vi "Error Query.vi"(8 "error in (no error)":errorcluster, 11 "VISA resource name":refnum<visa-resource-name>) -> (0 "error out":errorcluster, 1 "Error Message":string, 2 "Error Code":i32[](array[numeric]), 3 "VISA resource name out":refnum<visa-resource-name>)   [LabVIEW 2020, in "BDAQ-6104.lvlib"]
doc: "Queries the instrument for any errors in the instrument's error queue. It will continue to read errors until all errors have been read from the instrument. Any errors will be returned in the <B>error out</B> control.\n\n<B>Note:</B>\nThis VI is called automatically by most driver VIs so it is not usually necessary to call this in an application."
uses:
  <instrlib>/BDAQ-6104/BDAQ-6104.lvlib
panel:
  # "EDIT: Note: The Error Query VI is included as a subVI in all driver VIs except low-level API VIs. If the instrument does not support error query, then remove the VI and remove subVI calls in each instrument driver VI that calls it."
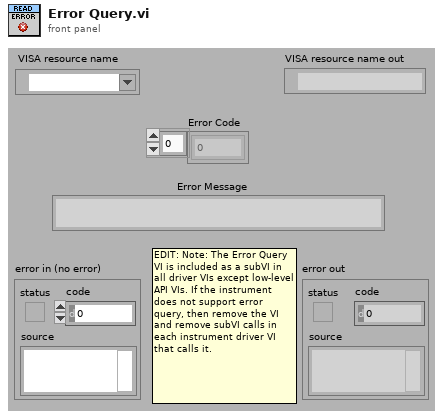
[diagram p1: front panel]
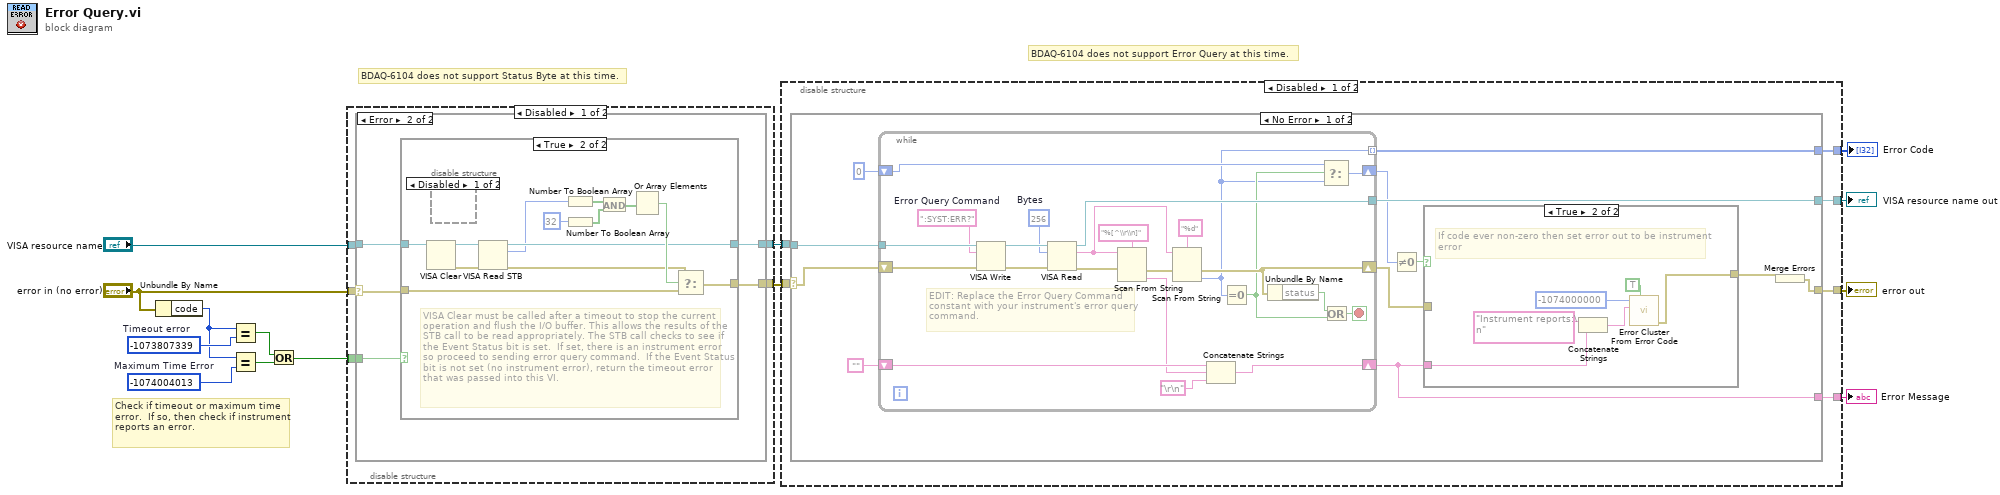
[diagram p0: block diagram]
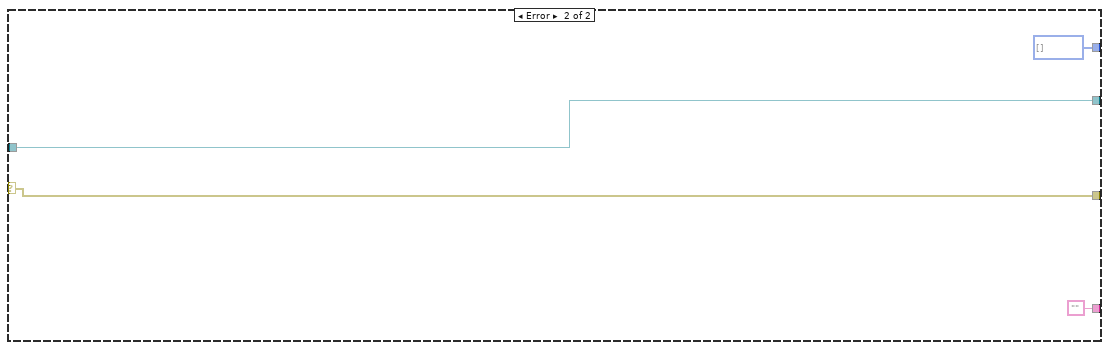
[diagram p7: hidden frame]
diagram:
  w5 = -1074004013  # Maximum Time Error
  w7 = -1073807339  # Timeout error
  # "BDAQ-6104 does not support Status Byte at this time."
  # "BDAQ-6104 does not support Error Query at this time."
  # "Check if timeout or maximum time error.  If so, then check if instrument reports an error."
  n1 = Unbundle By Name("error in (no error)") -> ("code"=w6:i32)
  n2 = Equal?(x=w6, y=w7) -> (x = y?=w3:bool)
  n3 = Equal?(x=w6, y=w5) -> (x = y?=w4:bool)
  n4 = Or(x=w3, y=w4) -> (x .or. y?=w2:bool)
  n5 = disable-structure shown="Disabled" {
    disable-tunnel: [w19 w42] -> w10
    disable-tunnel: [w18 w43] -> w9
    disable-tunnel: "VISA resource name" -> [w17 w43]
    disable-tunnel: w2 -> [w16 _]
    disable-tunnel: "error in (no error)" -> [w15 w42]
    frame Disabled {
      n6 = case shown="Error" w15 {
        selector: w15 -> [w20 w24]
        tunnel: w17 -> [w21 w26]
        tunnel: [w21 w25] -> w18
        tunnel: [w20 w23] -> w19
        tunnel: w16 -> [_ w22]
        frame No Error {
        }
        frame Error {
          n7 = case shown="True" w22 {
            tunnel: w26 -> [w28 w34]
            tunnel: [w28 w31] -> w25
            tunnel: w24 -> [w27 w37]
            tunnel: [w27 w36] -> w23
            frame False {
              # "Error code not a timeout, so best to pass on to user."
            }
            frame True {
              # "VISA Clear must be called after a timeout to stop the current operation and flush the I/O buffer. This allows the results of the  STB call to be read appropriately. The STB call checks to see if the Event Status bit is set.  If set, there is an instrument error so proceed to sending error query command.  If the Event Status bit is not set (no instrument error), return the timeout error that was passed into this VI."
              n8 = VISA Clear(VISA resource name=w34) -> (VISA resource name out=w33:refnum<visa-resource-name>, error out=w32:errorcluster)  [unwired: 1 in]
              n9 = disable-structure shown="Disabled" {
                frame Disabled {
                }
                frame Enabled {
                }
              }
              n10 = VISA Read STB(8:w32, 11:w33) -> (0:w30:errorcluster, 2:w29:u16, 3:w31:refnum<visa-resource-name>)
              n11 = Number To Boolean Array(number=w29) -> (Boolean array=w38:bool[])
              n12 = Number To Boolean Array(number=32) -> (Boolean array=w40:bool[])
              n13 = And(x=w38, y=w40) -> (x .and. y?=w39:bool[])
              n14 = Or Array Elements(Boolean array=w39) -> (logical OR=w35:bool)
              n15 = Select(t=w30, s=w35, f=w37) -> (s? t:f=w36:errorcluster)
            }
          }
        }
      }
    }
    frame Enabled {
    }
  }
  n16 = disable-structure shown="Disabled" {
    disable-tunnel: [w49 w97] -> w14
    disable-tunnel: [w48 w96] -> w13
    disable-tunnel: [w47 _] -> w12
    disable-tunnel: [w46 _] -> w11
    disable-tunnel: w10 -> [w45 w96]
    disable-tunnel: w9 -> [w44 w97]
    frame Disabled {
      n17 = case shown="No Error" w45 {
        selector: w45 -> [w50 w92]
        tunnel: [w61 w95] -> w49
        tunnel: w44 -> [w60 w95]
        tunnel: [w58 w92] -> w48
        tunnel: [w53 ""] -> w47
        tunnel: [w52 i32[] []] -> w46
        frame No Error {
          n18 = while {
            tunnel: [w91] -> w61
            tunnel: w60 -> [w90]
            shift-right: [w78] -> w53
            shift-left: "" -> [w81]
            shift-right: [w76] -> w54
            shift-left: 0 -> [w77]
            shift-right: [w74] -> w51
            shift-left: w50 -> [w75]
            tunnel: [w69] -> w52 mode=indexing
            stop <- w84 stop-if-true
            w88 = u32 256  # Bytes
            w86 = ":SYST:ERR?"  # Error Query Command
            # "EDIT: Replace the Error Query Command constant with your instrument's error query command."
            n19 = VISA Write(VISA resource name=w90, write buffer=w86, error in (no error)=w75) -> (VISA resource name out=w89:refnum<visa-resource-name>, error out=w87:errorcluster)  [unwired: 1 out]
            n20 = VISA Read(VISA resource name=w89, byte count=w88, error in (no error)=w87) -> (VISA resource name out=w91:refnum<visa-resource-name>, read buffer=w82:string, error out=w73:errorcluster)  [unwired: 1 out]
            n21 = Scan From String(format string="%[^\\r\\n]", input string=w82, error in=w73) -> (error out=w72:errorcluster, output 1=w79:string)  [unwired: 2 in, 2 out]
            n22 = Scan From String(format string="%d", input string=w82, error in=w72) -> (error out=w74:errorcluster, output 1=w69:i32)  [unwired: 2 in, 2 out]
            n23 = Concatenate Strings(w81, w79, "\r\n") -> (w78:string)
            n24 = Equal To 0?(x=w69) -> (x = 0?=w70:bool)
            n25 = Unbundle By Name(w74) -> ("status"=w71:bool)
            n26 = Select(t=w77, s=w70, f=w69) -> (s? t:f=w76:i32)
            n27 = Or(x=w71, y=w70) -> (x .or. y?=w84:bool)
          }
          n28 = Not Equal To 0?(x=w54) -> (x != 0?=w56:bool)
          n29 = case shown="True" w56 {
            tunnel: w53 -> [_ w67]
            tunnel: [w62 w63] -> w55
            tunnel: w51 -> [w62 _]
            frame False {
            }
            frame True {
              # "If code ever non-zero then set error out to be instrument error"
              n30 = Concatenate Strings("Instrument reports:\n" ("Source"), w67) -> (w64:string)
              n31 = call <vilib>:"Error Cluster From Error Code.vi"("show call chain? (False)"=TRUE, "error message (\"\")"=w64, "error code (0)"=-1074000000 ("Code")) -> ("error out"=w63:errorcluster)  [unwired: 6 in]
            }
          }
          n32 = Merge Errors(w55) -> (w58:errorcluster)
        }
        frame Error {
        }
      }
    }
    frame Enabled {
    }
  }
  "VISA resource name out" <- w14
  "error out" <- w13
  "Error Message" <- w12
  "Error Code" <- w11
